vi "Create Fan Controller.vi"(8 "error in (no error)":errorcluster, 11 "Fan Controller Type":refnum<class "iFan Controller.lvclass">) -> (0 "error out":errorcluster, 3 "Fan Controller Ref":refnum<data-value>)   [LabVIEW 2019, in "Fan Controller Ref.lvclass"]
uses:
  <vilib>/gpm_packages/@cs/Car-wash/Source/Fan Controller Ref/Fan Controller Ref.lvclass
  <vilib>/gpm_packages/@cs/Car-wash/Source/iFan Controller/iFan Controller.lvclass
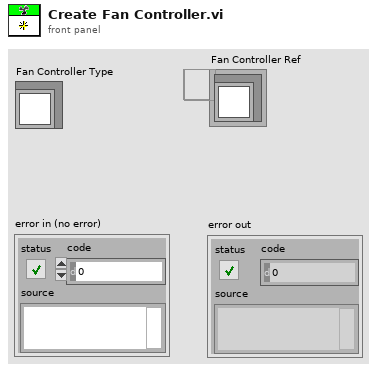
[diagram p1: front panel]
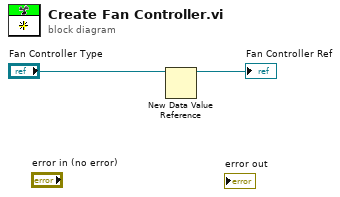
[diagram p0: block diagram]
diagram:
  n1 = New Data Value Reference(data value="Fan Controller Type") -> (data value reference=→"Fan Controller Ref":refnum<data-value>)  [unwired: 1 in, 1 out]
